vi "great.vi"() -> ()   [LabVIEW 2024]
panel:
  out "SMALL":dbl
  out "GREAT":dbl
  in  "C":dbl
  in  "B":dbl
  in  "A":dbl
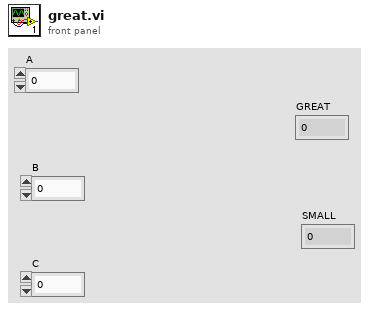
[diagram p1: front panel]
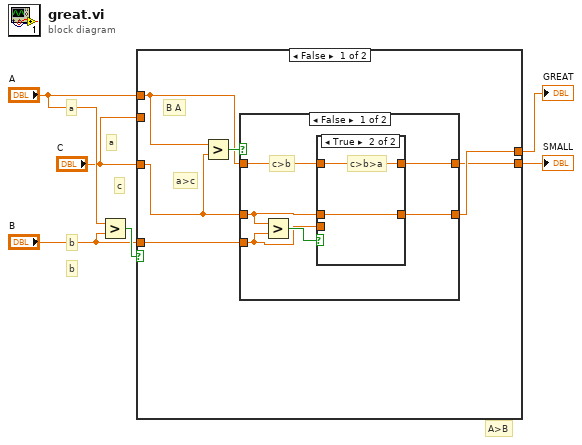
[diagram p0: block diagram]
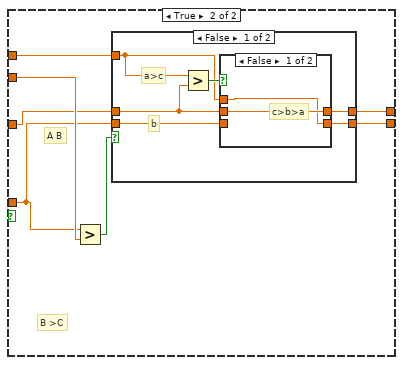
[diagram p4: hidden frame]
diagram:
  # "c"
  # "a"
  # "b"
  # "b"
  # "a"
  # "A>B"
  n1 = Greater?(x="A", y="B") -> (0:w6:bool)
  n2 = case shown="False" w6 {
    tunnel: "B" -> [w10 w25]
    tunnel: "C" -> [_ w31]
    tunnel: "A" -> [w7 w29]
    tunnel: "C" -> [w11 w28]
    tunnel: [w9 w27] -> w2
    tunnel: [w8 w26] -> w1
    frame False {
      # "a>c"
      # "B A"
      n3 = Greater?(x=w7, y=w11) -> (0:w12:bool)
      n4 = case shown="False" w12 {
        tunnel: w11 -> [w13 w23]
        tunnel: w10 -> [w17 w24]
        tunnel: [w16 w24] -> w9
        tunnel: [w14 w23] -> w8
        tunnel: w7 -> [w15 _]
        frame False {
          # "c>b"
          n5 = Greater?(x=w13, y=w17) -> (0:w18:bool)
          n6 = case shown="True" w18 {
            tunnel: w17 -> [w20 _]
            tunnel: [w20 w21] -> w16
            tunnel: w15 -> [w19 w22]
            tunnel: [w19 w22] -> w14
            tunnel: w13 -> [_ w21]
            frame False {
              # "b>c>a"
            }
            frame True {
              # "c>b>a"
            }
          }
        }
        frame True {
          # "b>a>c"
        }
      }
    }
    frame True {
      # "B >C"
      # "A B"
      n7 = Greater?(x=w25, y=w31) -> (0:w30:bool)
      n8 = case shown="False" w30 {
        tunnel: w29 -> [w36 w43]
        tunnel: w28 -> [w32 w42]
        tunnel: [w35 w43] -> w27
        tunnel: [w33 w42] -> w26
        tunnel: w25 -> [w34 _]
        frame False {
          # "b"
          # "a>c"
          n9 = Greater?(x=w36, y=w32) -> (0:w37:bool)
          n10 = case shown="False" w37 {
            tunnel: w36 -> [w38 w41]
            tunnel: [w39 w41] -> w35
            tunnel: w34 -> [_ w40]
            tunnel: [w38 w40] -> w33
            tunnel: w32 -> [w39 _]
            frame False {
              # "c>b>a"
            }
            frame True {
              # "a>c>b"
            }
          }
        }
        frame True {
          # "a b c"
        }
      }
    }
  }
  "GREAT" <- w2
  "SMALL" <- w1
